vi "fgv_gps-mode_history.vi"(7 "cmd":T2, 11 "data":T1) -> (3 "data out":T1)   [LabVIEW 2019]
uses:
  Ctrl/cmd_ini-RW.ctl
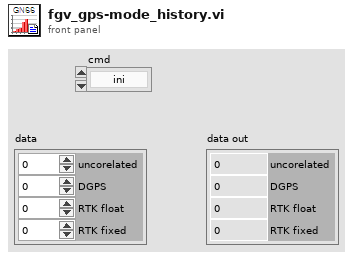
[diagram p1: front panel]
types:
  T1 = cluster{"uncorelated":u32, "DGPS":u32, "RTK float":u32, "RTK fixed":u32}
  T2 = typedef "cmd_ini-RW.ctl" = enum16{"ini", "read", "write"}
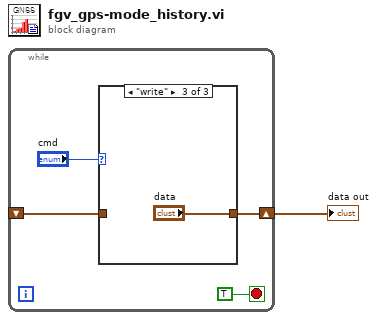
[diagram p0: block diagram]
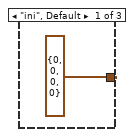
[diagram p2: hidden frame]
diagram:
  n1 = while {
    shift-right: [w3] -> w1
    shift-left: _ -> [w2]
    stop <- TRUE stop-if-true
    n2 = case shown="\"write\"" "cmd" {
      tunnel: [T1 {"uncorelated"=0, "DGPS"=0, "RTK float"=0, "RTK fixed"=0} ("data") w7 "data"] -> w3
      tunnel: w2 -> [_ w7 _]
      frame "ini", Default {
      }
      frame "read" {
      }
      frame "write" {
      }
    }
  }
  "data out" <- w1
